vi "Config - Load.vi"(8 "error in (no error)":errorcluster, 11 "Config Data":T1[](array[typedef]) {"Step Duration" max=99999 step=1}) -> (0 "error out":errorcluster, 3 "Config Data":T1[](array[typedef]) {"Step Duration" max=99999 step=1})   [LabVIEW 2017]
doc: "Provide full access to the configuration data records\n[Covers: SD6]"
uses:
  Controls/Congif Data.ctl
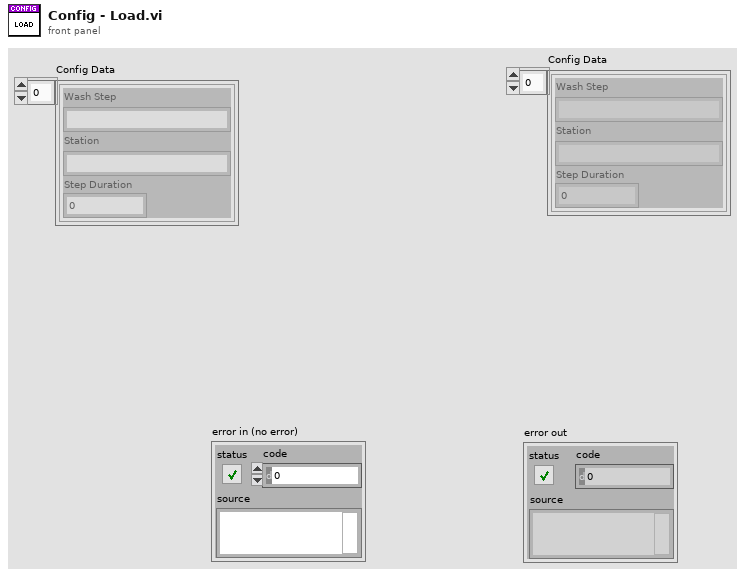
[diagram p1: front panel]
types:
  T1 = typedef "Congif Data.ctl" = cluster{"Wash Step":string, "Station":string, "Step Duration":u32}
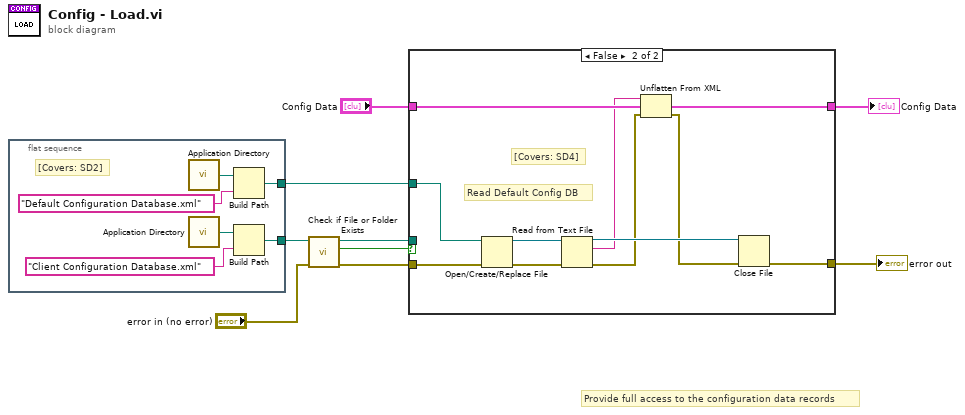
[diagram p0: block diagram]
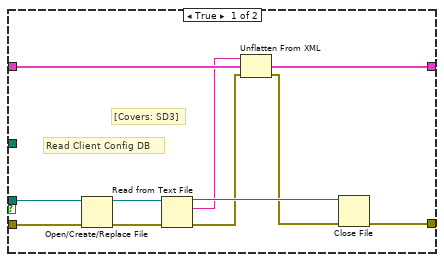
[diagram p2: hidden frame]
diagram:
  # "Provide full access to the configuration data records"
  n1 = flat-sequence {
    tunnel: [w13] -> w9
    tunnel: [w10] -> w4
    frame #0 {
      # "[Covers: SD2]"
      n2 = call <vilib>:"Application Directory.vi"() -> ("Application Directory"=w12:path)
      n3 = call <vilib>:"Application Directory.vi"() -> ("Application Directory"=w14:path)
      n4 = Build Path(base path=w12, name or relative path="Default Configuration Database.xml") -> (appended path=w10:path)
      n5 = Build Path(base path=w14, name or relative path="Client Configuration Database.xml") -> (appended path=w13:path)
    }
  }
  n6 = call <vilib>:"Check if File or Folder Exists.vi"("error in (no error)"="error in (no error)", "path"=w9) -> ("error out"=w5:errorcluster, "file or folder exists?"=w7:bool, "dup path"=w6:path)  [unwired: 7 in]
  n7 = case shown="False" w7 {
    tunnel: w6 -> [w20 _]
    tunnel: w5 -> [w21 w32]
    tunnel: w4 -> [_ w29]
    tunnel: "Config Data" -> [w19 w31]
    tunnel: [w17 w28] -> w3
    tunnel: [w16 w27] -> w1
    frame True {
      # "Read Client Config DB"
      # "[Covers: SD3]"
      n8 = Open/Create/Replace File(file path (use dialog)=w20, error in=w21) -> (refnum out=w23:refnum<file>, error out=w22:errorcluster)  [unwired: 4 in, 1 out]
      n9 = Read from Text File(file (use dialog)=w23, error in=w22) -> (refnum out=w26:refnum<file>, text=w18:string, error out=w24:errorcluster)  [unwired: 2 in, 1 out]
      n10 = Unflatten From XML(xml string=w18, type=w19, error in (no error)=w24) -> (value=w16:T1[], error out=w25:errorcluster)
      n11 = Close File(refnum=w26, error in=w25) -> (error out=w17:errorcluster)  [unwired: 1 out]
    }
    frame False {
      # "Read Default Config DB"
      # "[Covers: SD4]"
      n12 = Open/Create/Replace File(file path (use dialog)=w29, error in=w32) -> (refnum out=w34:refnum<file>, error out=w33:errorcluster)  [unwired: 4 in, 1 out]
      n13 = Read from Text File(file (use dialog)=w34, error in=w33) -> (refnum out=w37:refnum<file>, text=w30:string, error out=w35:errorcluster)  [unwired: 2 in, 1 out]
      n14 = Unflatten From XML(xml string=w30, type=w31, error in (no error)=w35) -> (value=w27:T1[], error out=w36:errorcluster)
      n15 = Close File(refnum=w37, error in=w36) -> (error out=w28:errorcluster)  [unwired: 1 out]
    }
  }
  "error out" <- w3
  "Config Data" <- w1
